vi "Constants.vi"(2 "Cluster 2":cluster{string, i32}, 3 "Cluster":cluster{string, i32}) -> ()   [LabVIEW 2017]
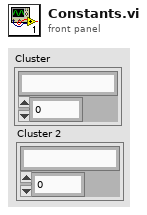
[diagram p1: front panel]
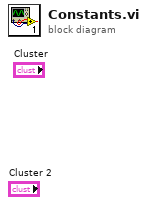
[diagram p0: block diagram]
diagram:
